vi "TimeWizard_NoSearch.vi"(0 "Time/Date Format":string(combo)="%I:%M %p\\n%d-%b-%y", 1 "Select Time Zone":u32(ring)=142 items=["Abbreviation (Time Zone Name)", "A (Alpha Time Zone)", "ACDT (Australian Central Daylight Time  CDT – Central Daylight Time CDST – Central Daylight Savings Time)", "ACST (Australian Central Standard Time  CST – Central Standard Time)", "ACT (Acre Time)", "ACT (Australian Central Time)", "ACWST (Australian Central Western Standard Time)", "ADT (Arabia Daylight Time  AST – Arabia Summer Time)", "ADT (Atlantic Daylight Time  ADST – Atlantic Daylight Saving Time AST – Atlantic Summer Time  HAA – Heure Avancée de l'Atlantique (French))", "AEDT (Australian Eastern Daylight Time  EDT – Eastern Daylight Time EDST – Eastern Daylight Saving Time)", "AEST (Australian Eastern Standard Time  EST – Eastern Standard Time AET – Australian Eastern Time)", "AET (Australian Eastern Time)", "AFT (Afghanistan Time)", "AKDT (Alaska Daylight Time  ADST – Alaska Daylight Saving Time)", "AKST (Alaska Standard Time  AT – Alaska Time)", "ALMT (Alma-Ata Time)", "AMST (Amazon Summer Time)", "AMST (Armenia Summer Time  AMDT – Armenia Daylight Time)", "AMT (Amazon Time)", "AMT (Armenia Time)", "ANAST (Anadyr Summer Time)", "ANAT (Anadyr Time)", "AQTT (Aqtobe Time)", "ART (Argentina Time)", "AST (Arabia Standard Time  AST – Arabic Standard Time AST – Al Manamah Standard Time)", "AST (Atlantic Standard Time  AT – Atlantic Time  AST – Tiempo Estándar del Atlántico (Spanish) HNA – Heure Normale de l'Atlantique (French))", "AT (Atlantic Time)", "AWDT (Australian Western Daylight Time  WDT – Western Daylight Time WST – Western Summer Time)", "AWST (Australian Western Standard Time  WST – Western Standard Time WAT – Western Australia Time)", "AZOST (Azores Summer Time  AZODT – Azores Daylight Time)", "AZOT (Azores Time  AZOST – Azores Standard Time)", "AZST (Azerbaijan Summer Time)", "AZT (Azerbaijan Time)", "AoE (Anywhere on Earth)", "B (Bravo Time Zone)", "BNT (Brunei Darussalam Time  BDT – Brunei Time)", "BOT (Bolivia Time)", "BRST (Brasília Summer Time  BST – Brazil Summer Time BST – Brazilian Summer Time)", "BRT (Brasília Time  BT – Brazil Time BT – Brazilian Time)", "BST (Bangladesh Standard Time)", "BST (Bougainville Standard Time)", "BST (British Summer Time  BDT – British Daylight Time BDST – British Daylight Saving Time)", "BTT (Bhutan Time)", "C (Charlie Time Zone)", "CAST (Casey Time)", "CAT (Central Africa Time)", "CCT (Cocos Islands Time)", "CDT (Central Daylight Time  CDST – Central Daylight Saving Time NACDT – North American Central Daylight Time  HAC – Heure Avancée du Centre (French))", "CDT (Cuba Daylight Time)", "CEST (Central European Summer Time  CEDT – Central European Daylight Time ECST – European Central Summer Time  MESZ – Mitteleuropäische Sommerzeit (German))", "CET (Central European Time  ECT – European Central Time CET – Central Europe Time  MEZ – Mitteleuropäische Zeit (German))", "CHADT (Chatham Island Daylight Time  CDT – Chatham Daylight Time)", "CHAST (Chatham Island Standard Time)", "CHOST (Choibalsan Summer Time  CHODT – Choibalsan Daylight Time CHODST – Choibalsan Daylight Saving Time)", "CHOST (Choibalsan Summer Time)", "CHOT (Choibalsan Time)", "CHUT (Chuuk Time)", "CIDST (Cayman Islands Daylight Saving Time)", "CIST (Cayman Islands Standard Time  CIT – Cayman Islands Time)", "CKT (Cook Island Time)", "CLST (Chile Summer Time  CLDT – Chile Daylight Time)", "CLT (Chile Standard Time  CT – Chile Time CLST – Chile Standard Time)", "COT (Colombia Time)", "CST (Central Standard Time  CT – Central Time NACST – North American Central Standard Time  CST – Tiempo Central Estándar (Spanish) HNC – Heure Normale du Centre (French))", "CST (China Standard Time)", "CST (Cuba Standard Time)", "CT (Central Time)", "CVT (Cape Verde Time)", "CXT (Christmas Island Time)", "ChST (Chamorro Standard Time  GST – Guam Standard Time)", "D (Delta Time Zone)", "DAVT (Davis Time)", "DDUT (Dumont-d'Urville Time)", "E (Echo Time Zone)", "EASST (Easter Island Summer Time  EADT – Easter Island Daylight Time)", "EAST (Easter Island Standard Time)", "EAT (Eastern Africa Time  EAT – East Africa Time)", "ECT (Ecuador Time)", "EDT (Eastern Daylight Time  EDST – Eastern Daylight Savings Time NAEDT – North American Eastern Daylight Time  HAE – Heure Avancée de l'Est (French) EDT – Tiempo de verano del Este (Spanish))", "EEST (Eastern European Summer Time  EEDT – Eastern European Daylight Time  OESZ – Osteuropäische Sommerzeit (German))", "EET (Eastern European Time  OEZ – Osteuropäische Zeit (German))", "EGST (Eastern Greenland Summer Time  EGST – East Greenland Summer Time)", "EGT (East Greenland Time  EGT – Eastern Greenland Time)", "EST (Eastern Standard Time  ET – Eastern Time  NAEST – North American Eastern Standard Time  ET – Tiempo del Este (Spanish) HNE – Heure Normale de l'Est (French))", "ET (Eastern Time)", "F (Foxtrot Time Zone)", "FET (Further-Eastern European Time)", "FJST (Fiji Summer Time  FJDT – Fiji Daylight Time)", "FJT (Fiji Time)", "FKST (Falkland Islands Summer Time  FKDT – Falkland Island Daylight Time)", "FKT (Falkland Island Time  FKST – Falkland Island Standard Time)", "FNT (Fernando de Noronha Time)", "G (Golf Time Zone)", "GALT (Galapagos Time)", "GAMT (Gambier Time  GAMT – Gambier Islands Time)", "GET (Georgia Standard Time)", "GFT (French Guiana Time)", "GILT (Gilbert Island Time)", "GMT (Greenwich Mean Time  \"– Coordinated Universal Time GT – Greenwich Time)", "GST (Gulf Standard Time)", "GST (South Georgia Time)", "GYT (Guyana Time)", "H (Hotel Time Zone)", "HADT (Hawaii-Aleutian Daylight Time  HDT – Hawaii Daylight Time)", "HAST (Hawaii-Aleutian Standard Time  HST – Hawaii Standard Time)", "HKT (Hong Kong Time)", "HOVST (Hovd Summer Time  HOVDT – Hovd Daylight Time HOVDST – Hovd Daylight Saving Time)", "HOVST (Hovd Summer Time)", "HOVT (Hovd Time)", "I (India Time Zone)", "ICT (Indochina Time)", "IDT (Israel Daylight Time)", "IOT (Indian Chagos Time)", "IRDT (Iran Daylight Time  IRST – Iran Summer Time IDT – Iran Daylight Time)", "IRKST (Irkutsk Summer Time)", "IRKT (Irkutsk Time)", "IRST (Iran Standard Time  IT – Iran Time)", "IST (India Standard Time  IT – India Time IST – Indian Standard Time)", "IST (Irish Standard Time  IST – Irish Summer Time)", "IST (Israel Standard Time)", "JST (Japan Standard Time)", "K (Kilo Time Zone)", "KGT (Kyrgyzstan Time)", "KOST (Kosrae Time)", "KRAST (Krasnoyarsk Summer Time)", "KRAT (Krasnoyarsk Time)", "KST (Korea Standard Time  KST – Korean Standard Time KT – Korea Time)", "KUYT (Kuybyshev Time  SAMST – Samara Summer Time)", "L (Lima Time Zone)", "LHDT (Lord Howe Daylight Time)", "LHST (Lord Howe Standard Time)", "LINT (Line Islands Time)", "M (Mike Time Zone)", "MAGST (Magadan Summer Time  MAGST – Magadan Island Summer Time)", "MAGT (Magadan Time  MAGT – Magadan Island Time)", "MART (Marquesas Time)", "MAWT (Mawson Time)", "MDT (Mountain Daylight Time  MDST – Mountain Daylight Saving Time NAMDT – North American Mountain Daylight Time  HAR – Heure Avancée des Rocheuses (French))", "MHT (Marshall Islands Time)", "MMT (Myanmar Time)", "MSD (Moscow Daylight Time  Moscow Summer Time)", "MSK (Moscow Standard Time  MCK – Moscow Time)", "MST (Mountain Standard Time  MT – Mountain Time NAMST – North American Mountain Standard Time  HNR – Heure Normale des Rocheuses (French))", "MT (Mountain Time)", "MUT (Mauritius Time)", "MVT (Maldives Time)", "MYT (Malaysia Time  MST – Malaysian Standard Time)", "N (November Time Zone)", "NCT (New Caledonia Time)", "NDT (Newfoundland Daylight Time  HAT – Heure Avancée de Terre-Neuve (French))", "NFT (Norfolk Time  NFT – Norfolk Island Time)", "NOVST (Novosibirsk Summer Time  OMSST – Omsk Summer Time)", "NOVT (Novosibirsk Time  OMST – Omsk Standard Time)", "NPT (Nepal Time)", "NRT (Nauru Time)", "NST (Newfoundland Standard Time  HNT – Heure Normale de Terre-Neuve (French))", "NUT (Niue Time)", "NZDT (New Zealand Daylight Time)", "NZST (New Zealand Standard Time)", "O (Oscar Time Zone)", "OMSST (Omsk Summer Time  NOVST – Novosibirsk Summer Time)", "OMST (Omsk Standard Time  OMST – Omsk Time NOVT – Novosibirsk Time)", "ORAT (Oral Time)", "P (Papa Time Zone)", "PDT (Pacific Daylight Time  PDST – Pacific Daylight Saving Time NAPDT – North American Pacific Daylight Time  HAP – Heure Avancée du Pacifique (French))", "PET (Peru Time)", "PETST (Kamchatka Summer Time)", "PETT (Kamchatka Time  PETT – Petropavlovsk-Kamchatski Time)", "PGT (Papua New Guinea Time)", "PHOT (Phoenix Island Time)", "PHT (Philippine Time  PST – Philippine Standard Time)", "PKT (Pakistan Standard Time  PKT – Pakistan Time)", "PMDT (Pierre & Miquelon Daylight Time)", "PMST (Pierre & Miquelon Standard Time)", "PONT (Pohnpei Standard Time)", "PST (Pacific Standard Time  PT – Pacific Time NAPST – North American Pacific Standard Time  PT – Tiempo del Pacífico (Spanish) HNP – Heure Normale du Pacifique (French))", "PST (Pitcairn Standard Time)", "PT (Pacific Time)", "PWT (Palau Time)", "PYST (Paraguay Summer Time)", "PYT (Paraguay Time)", "PYT (Pyongyang Time  PYST – Pyongyang Standard Time)", "PYT (Pyongyang Time)", "Q (Quebec Time Zone)", "QYZT (Qyzylorda Time)", "R (Romeo Time Zone)", "RET (Reunion Time)", "ROTT (Rothera Time)", "S (Sierra Time Zone)", "SAKT (Sakhalin Time)", "SAMT (Samara Time  SAMT – Samara Standard Time)", "SAST (South Africa Standard Time  SAST – South African Standard Time)", "SBT (Solomon Islands Time  SBT – Solomon Island Time)", "SCT (Seychelles Time)", "SGT (Singapore Time  SST – Singapore Standard Time)", "SRET (Srednekolymsk Time)", "SRT (Suriname Time)", "SST (Samoa Standard Time)", "SYOT (Syowa Time)", "T (Tango Time Zone)", "TAHT (Tahiti Time)", "TFT (French Southern and Antarctic Time  KIT – Kerguelen (Islands) Time)", "TJT (Tajikistan Time)", "TKT (Tokelau Time)", "TLT (East Timor Time)", "TMT (Turkmenistan Time)", "TOT (Tonga Time)", "TVT (Tuvalu Time)", "U (Uniform Time Zone)", "ULAST (Ulaanbaatar Summer Time  ULAST – Ulan Bator Summer Time)", "ULAST (Ulaanbaatar Summer Time)", "ULAT (Ulaanbaatar Time  ULAT – Ulan Bator Time)", "ULAT (Ulaanbaatar Time)", "UTC (Coordinated Universal Time)", "UYST (Uruguay Summer Time)", "UYT (Uruguay Time)", "UZT (Uzbekistan Time)", "V (Victor Time Zone)", "VET (Venezuelan Standard Time  HLV – Hora Legal de Venezuela (Spanish))", "VLAST (Vladivostok Summer Time)", "VLAT (Vladivostok Time)", "VOST (Vostok Time)", "VUT (Vanuatu Time  EFATE – Efate Time)", "W (Whiskey Time Zone)", "WAKT (Wake Time)", "WARST (Western Argentine Summer Time)", "WAST (West Africa Summer Time)", "WAT (West Africa Time)", "WEST (Western European Summer Time  WEDT – Western European Daylight Time  WESZ – Westeuropäische Sommerzeit (German))", "WET (Western European Time  GMT – Greenwich Mean Time  WEZ – Westeuropäische Zeit (German))", "WFT (Wallis and Futuna Time)", "WGST (Western Greenland Summer Time  WGST – West Greenland Summer Time)", "WGT (West Greenland Time  WGT – Western Greenland Time)", "WIB (Western Indonesian Time  WIB – Waktu Indonesia Barat)", "WIT (Eastern Indonesian Time  WIT – Waktu Indonesia Timur)", "WITA (Central Indonesian Time  WITA – Waktu Indonesia Tengah)", "WST (West Samoa Time  ST – Samoa Time)", "WST (Western Sahara Summer Time)", "WT (Western Sahara Standard Time  WT – Western Sahara Time)", "X (X-ray Time Zone)", "Y (Yankee Time Zone)", "YAKST (Yakutsk Summer Time)", "YAKT (Yakutsk Time)", "YAPT (Yap Time)", "YEKST (Yekaterinburg Summer Time)", "YEKT (Yekaterinburg Time)", "Z (Zulu Time Zone)"]) -> (3 "Format String":string="%I:%M %p\\n%d-%b-%y", 4 "Formatted date/time string":string="05:00 PM\\n21-Jan-16", 5 "TZ Shift (hrs)":string="UTC-7.00", 6 "TZ Shift (sec)":dbl=-25200.0 format="%#_6f")   [LabVIEW 2022 SP3]
panel:
  in  "stop":bool
  out "Locale Time Stamp":timestamp=timestamp(3536265609.732094 s since 1904-01-01) format="%<%I:%M:%S %p\n%m/%d/%y>T"
  out "UTC Time Stamp":timestamp=timestamp(3536290809.732094 s since 1904-01-01) format="%<%I:%M:%S %p\n%m/%d/%y>T"
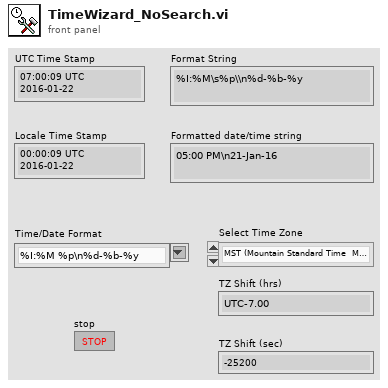
[diagram p1: front panel]
types:
  T1 = enum32{"Bad", "Idle", "Run top level", "Running"}
  T2 = typedef "LVDateTimeRec.ctl" = cluster{"fractional second":dbl, "second":i32, "minute":i32, "hour":i32, "day of month":i32, "month":i32, "year":i32, "day of week":i32, "day of year":i32, "DST":i32}
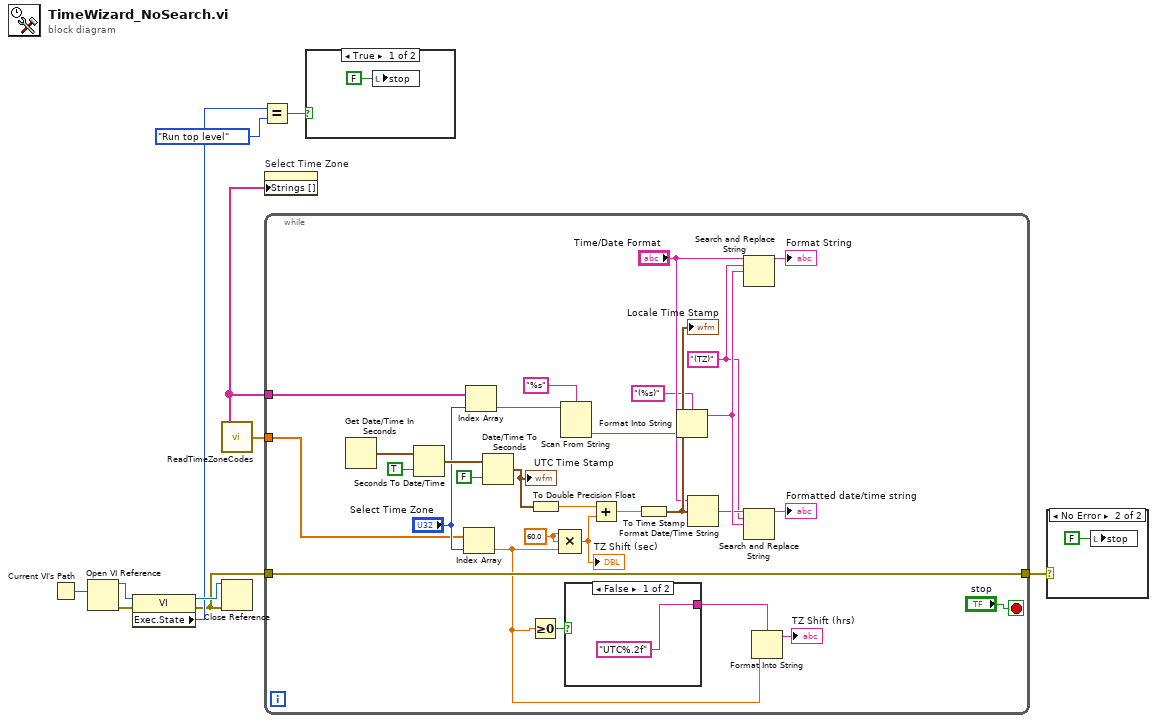
[diagram p0: block diagram]
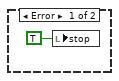
[diagram p2: hidden frame]
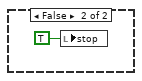
[diagram p3: hidden frame]
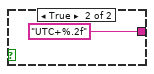
[diagram p4: hidden frame]
diagram:
  n1 = Current VI's Path() -> (path=w11:path)
  n2 = Open VI Reference(vi path=w11) -> (vi reference=w10:refnum<vi>, error out=w9:errorcluster)  [unwired: 5 in]
  n3 = property class="VI"(reference=w10, error in=w9) -> (reference out=w8:refnum<vi>, error out=w4:errorcluster, "Exec.State"=w7:T1)
  n4 = call "ReadTimeZoneCodes.vi"() -> ("x+y"=w2:dbl[], "Abbreviation"=w1:string[])
  n5 = Close Reference(reference=w8, error in (no error)=w4) -> ()  [unwired: 1 out]
  n6 = Equal?(x=w7, y=T1."Run top level" ("Execution:State 2")) -> (x = y?=w5:bool)
  n7 = property on="Select Time Zone" class="Ring (strict)"("Strings []"=w1) -> ()  [unwired: 2 in, 2 out]
  n8 = while {
    tunnel: w4 -> [w29]
    tunnel: [w29] -> w3
    tunnel: w2 -> [w24]
    tunnel: w1 -> [w23]
    stop <- "stop" stop-if-true
    w16 = "(TZ)" ("search string")
    w40 = 60.0 ("value")
    n9 = Get Date/Time In Seconds() -> (seconds since 1Jan1904=w33:timestamp)
    n10 = Seconds To Date/Time(time stamp (now)=w33, to UTC (F)=TRUE) -> (date time rec=w34:T2)
    n11 = Index Array(array=w24, index="Select Time Zone") -> (element=w12:dbl)
    n12 = Index Array(array=w23, index="Select Time Zone") -> (element=w26:string)
    n13 = Date/Time To Seconds(1:FALSE ("is UTC (F)"), 2:w34) -> (0:w32:timestamp)
    "UTC Time Stamp" <- w32
    n14 = Greater Or Equal To 0?(x=w12) -> (x >= 0?=w13:bool)
    n15 = To Double Precision Float(number=w32) -> (double precision float=w39:dbl)
    n16 = Compound Arithmetic op=MULTIPLY(w40, w40, w12) -> (w28:dbl)
    "TZ Shift (sec)" <- w28
    n17 = Scan From String(format string="%s", input string=w26) -> (output 1=w18:string)  [unwired: 3 in, 3 out]
    n18 = case shown="False" w13 {
      tunnel: ["UTC%.2f" ("format string") "UTC+%.2f" ("format string")] -> w15
      frame False {
      }
      frame True {
      }
    }
    n19 = Add(x=w39, y=w28) -> (x+y=w38:dbl)
    n20 = To Time Stamp(1:w38) -> (0:w30:timestamp)
    "Locale Time Stamp" <- w30
    n21 = Format Into String(format string="(%s)", w18) -> (resulting string=w25:string)  [unwired: 2 in, 1 out]
    n22 = Format Date/Time String(time format string (%c)="Time/Date Format", seconds (now)=w30) -> (date/time string=w21:string)  [unwired: 1 in]
    n23 = Search and Replace String(input string="Time/Date Format", search string=w16, replace string=w25) -> (result string=→"Format String":string)  [unwired: 5 in, 3 out]
    n24 = Search and Replace String(input string=w21, search string=w16, replace string=w25) -> (result string=→"Formatted date/time string":string)  [unwired: 5 in, 3 out]
    n25 = Format Into String(format string=w15, w12) -> (resulting string=→"TZ Shift (hrs)":string)  [unwired: 2 in, 1 out]
  }
  n26 = case shown="True" w5 {
    frame True {
      n27 = local write "stop"(FALSE) -> ()
    }
    frame False {
      n28 = local write "stop"(TRUE) -> ()
    }
  }
  n29 = case shown="No Error" w3 {
    frame Error {
      n30 = local write "stop"(TRUE) -> ()
    }
    frame No Error {
      n31 = local write "stop"(FALSE) -> ()
    }
  }
